vi "Keith 7001 Arm Lay 1 Config.vi"(1 "count value":u16=1 min=1 max=9999, 2 "count":bool=TRUE, 3 "source bypass":bool, 4 "source (immediate:1)":u16(ring)=1 items=["hold", "immediate", "manual", "GPIB", "trigger link", "external"], 5 "error in":T1, 6 "trigger link output":u16=2 min=1 max=6 step=1, 7 "trigger link input":u16=1 min=1 max=6 step=1, 8 "GPIB address":string="7") -> (0 "error out":T1)   [LabVIEW 2019]
doc: "This VI for the Keithley 7001 Switch System configures arm layer 1 (arm layer)."
panel:
  # "enable (source)\ndisable (acceptor)"
  # "set finite value\ninfinite"
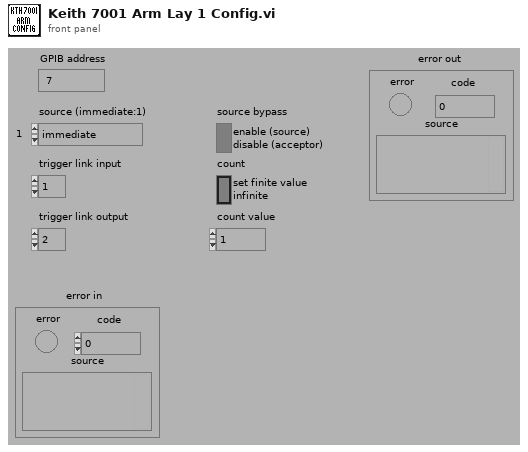
[diagram p1: front panel]
types:
  T1 = cluster{"error":bool, "code":i32, "source":string}
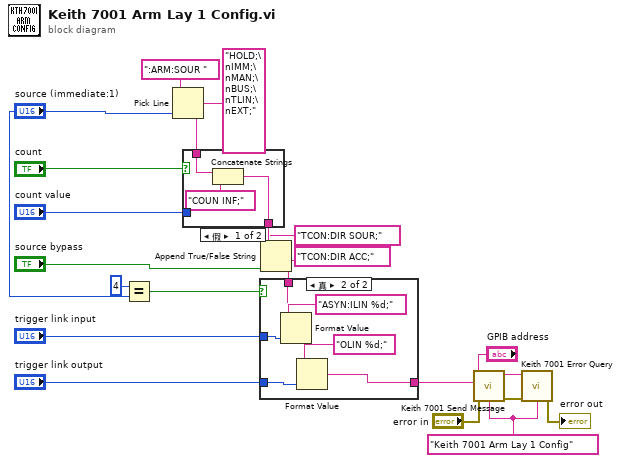
[diagram p0: block diagram]
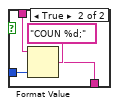
[diagram p3: hidden frame]
diagram:
  w2 = "Keith 7001 Arm Lay 1 Config"
  n1 = Equal?(x=4, y="source (immediate:1)") -> (x = y?=w10:bool)
  n2 = Pick Line(string ("")=":ARM:SOUR ", multi-line string="HOLD;\nIMM;\nMAN;\nBUS;\nTLIN;\nEXT;", line index="source (immediate:1)") -> (output string=w20:string)
  n3 = case shown="假" "count" {
    tunnel: w20 -> [w25 w29]
    tunnel: [w23 w26] -> w18
    tunnel: "count value" -> [_ w28]
    frame False {
      n4 = Concatenate Strings(w25, "COUN INF;") -> (w23:string)
    }
    frame True {
      n5 = Format Value(string ("")=w29, format string="COUN %d;", value (0)=w28) -> (output string=w26:string)
    }
  }
  n6 = Append True/False String(1:"source bypass", 2:"TCON:DIR ACC;", 3:"TCON:DIR SOUR;", 4:w18) -> (0:w13:string)
  n7 = case shown="真" w10 {
    tunnel: w13 -> [w30 w34]
    tunnel: [w30 w33] -> w12
    tunnel: "trigger link input" -> [_ w32]
    tunnel: "trigger link output" -> [_ w31]
    frame False {
    }
    frame True {
      n8 = Format Value(string ("")=w34, format string="ASYN:ILIN %d;", value (0)=w32) -> (output string=w36:string)
      n9 = Format Value(string ("")=w36, format string="OLIN %d;", value (0)=w31) -> (output string=w33:string)
    }
  }
  n10 = call "Keith 7001 Send Message.vi"("address string"="GPIB address", "write buffer"=w12, "source"=w2, "error in"="error in") -> ("address out"=w4:string, "error out"=w3:T1)  [unwired: 2 in, 2 out]
  n11 = call "Keith 7001 Error Query.vi"("GPIB address"=w4, "error in"=w3, "source"=w2) -> ("error out"=→"error out":T1)  [unwired: 2 out]
